vi "selectCursorProperties.vi"(6 "Cursor Properties in":T1={"Horizontal Line?"=TRUE, "Vertical Line?"=TRUE, "Timestamp"=enum."at BOTTOM", "time format (%H:%M:%S)"="%H:%M:%S", "size"=2, "font"={"Font Name"="Arial", "Size"=16, "Strikeout?"=FALSE, "Italic?"=FALSE, "Underline?"=FALSE, "Outline?"=FALSE, "Shadow"=FALSE, "Bold?"=FALSE}, "alignment(left, top)"={"Horizontal"=enum."center", "Vertical"=enum."center"}, "TextFormat"="%3$s\\n%2$.2f"} {"size" min=1 max=50}) -> (2 "ok":bool, 4 "Cursor Properties out":T1={"Horizontal Line?"=TRUE, "Vertical Line?"=TRUE, "Timestamp"=enum."at BOTTOM", "time format (%H:%M:%S)"="%H:%M:%S", "size"=2, "font"={"Font Name"="Arial", "Size"=16, "Strikeout?"=FALSE, "Italic?"=FALSE, "Underline?"=FALSE, "Outline?"=FALSE, "Shadow"=FALSE, "Bold?"=FALSE}, "alignment(left, top)"={"Horizontal"=enum."center", "Vertical"=enum."center"}, "TextFormat"="%3$s\\n%2$.2f"} {"size" min=1 max=50})   [LabVIEW 2017, in "QControl_Graph.lvclass"]
uses:
  QControl_Graph.lvclass
  Cursor Properties.ctl
  Font.ctl
  Alignment.ctl
  Alignment.Horizontal.ctl
  Alignment.Vertical.ctl
panel:
  in  "Y Label Vertical:":T5=enum."center"
  in  "Y Label Horizontal:":T4=enum."center"
  in  "Show Horizontal Lines":bool=TRUE
  in  "Show Vertical Lines":bool=TRUE
  in  "X Label Position:":enum16{"at TOP", "at BOTTOM", "none"}(ring)=enum."at BOTTOM"
  in  "Point Size:":i16=2 min=1 max=50
  in  "Time Format:":string
  in  "Name Format:":string
  in  "Bold":bool
  in  "Shadow":bool
  in  "Outline":bool
  in  "Strikeout":bool
  in  "Underline":bool
  in  "Italic":bool
  in  "Size :":i16
  in  "Font:":string
  in  "Cancel":bool
  in  "OK":bool
  # "Font"
  # "Effects"
  # "Cursor"
  # "Grid"
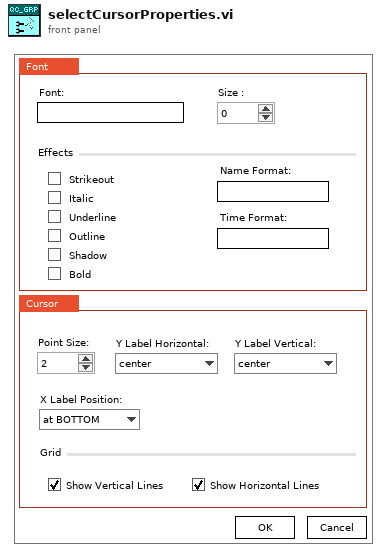
[diagram p1: front panel]
types:
  T1 = typedef "QControl_Graph.lvclass/Cursor Properties.ctl" = cluster{"Horizontal Line?":bool, "Vertical Line?":bool, "Timestamp":enum16{"at TOP", "at BOTTOM", "none"}, "time format (%H:%M:%S)":string, "size":i16, "font":T2, "alignment(left, top)":T3, "TextFormat":string}
  T2 = typedef "QControl_Graph.lvclass/Font.ctl" = cluster{"Font Name":string, "Size":i16, "Strikeout?":bool, "Italic?":bool, "Underline?":bool, "Outline?":bool, "Shadow":bool, "Bold?":bool}
  T3 = typedef "QControl_Graph.lvclass/Alignment.ctl" = cluster{"Horizontal":T4, "Vertical":T5}
  T4 = typedef "QControl_Graph.lvclass/Alignment.Horizontal.ctl" = enum16{"left", "center", "right"}
  T5 = typedef "QControl_Graph.lvclass/Alignment.Vertical.ctl" = enum16{"top", "center", "bottom"}
  T6 = enum32{"Invalid", "Standard", "Closed", "Hidden", "Minimized", "Maximized"}
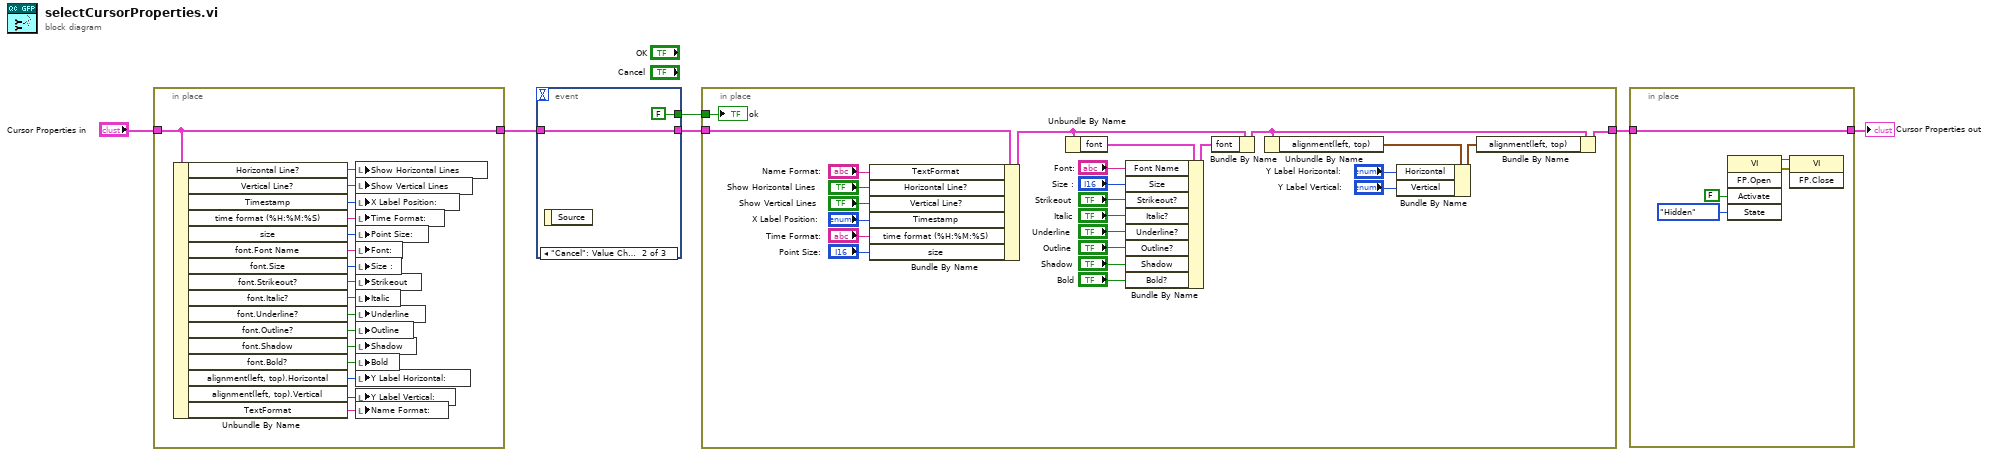
[diagram p0: block diagram]
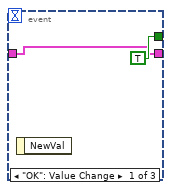
[diagram p2: hidden frame]
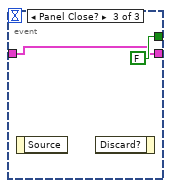
[diagram p3: hidden frame]
diagram:
  n1 = in-place {
    in-place-border: "Cursor Properties in" -> [w7]
    in-place-border: [w7] -> w5
    n2 = Unbundle By Name(w7) -> ("Horizontal Line?"=w23:bool, "Vertical Line?"=w22:bool, "Timestamp"=w21:enum16{"at TOP", "at BOTTOM", "none"}, "time format (%H:%M:%S)"=w20:string, "size"=w18:i16, "font.Font Name"=w19:string, "font.Size"=w17:i16, "font.Strikeout?"=w16:bool, "font.Italic?"=w8:bool, "font.Underline?"=w9:bool, "font.Outline?"=w10:bool, "font.Shadow"=w11:bool, "font.Bold?"=w12:bool, "alignment(left, top).Horizontal"=w15:T4, "alignment(left, top).Vertical"=w14:T5, "TextFormat"=w13:string)
    n3 = local write "Show Horizontal Lines"(w23) -> ()
    n4 = local write "Show Vertical Lines"(w22) -> ()
    n5 = local write "X Label Position:"(w21) -> ()
    n6 = local write "Time Format:"(w20) -> ()
    n7 = local write "Point Size:"(w18) -> ()
    n8 = local write "Font:"(w19) -> ()
    n9 = local write "Size :"(w17) -> ()
    n10 = local write "Strikeout"(w16) -> ()
    n11 = local write "Italic"(w8) -> ()
    n12 = local write "Underline"(w9) -> ()
    n13 = local write "Outline"(w10) -> ()
    n14 = local write "Shadow"(w11) -> ()
    n15 = local write "Bold"(w12) -> ()
    n16 = local write "Y Label Horizontal:"(w15) -> ()
    n17 = local write "Y Label Vertical:"(w14) -> ()
    n18 = local write "Name Format:"(w13) -> ()
  }
  n19 = event shown="[1] \"Cancel\": Value Change" {
    selector: _ -> [_ _ _]
    dyn-events: _ -> [_ _ _]
    timeout: _ -> [_ _ _]
    tunnel: [TRUE FALSE FALSE] -> w3
    tunnel: w5 -> [w24 w26 w28]
    tunnel: [w24 w26 w28] -> w4
    event "OK": Value Change {
      n20 = event-data() -> ()  [unwired: 1 in, 1 out]
    }
    event "Cancel": Value Change {
      n21 = event-data() -> ()  [unwired: 1 in, 1 out]
    }
    event Panel Close? {
      n22 = event-data() -> ()  [unwired: 1 in, 1 out]
      n23 = event-data() -> ()  [unwired: 2 in, 1 out]
    }
  }
  n24 = in-place {
    in-place-border: w4 -> [w48]
    in-place-border: [w31] -> w2
    in-place-border: w3 -> [w30]
    n25 = Bundle By Name(cluster=w48, "TextFormat"="Name Format:", "Horizontal Line?"="Show Horizontal Lines", "Vertical Line?"="Show Vertical Lines", "Timestamp"="X Label Position:", "time format (%H:%M:%S)"="Time Format:", "size"="Point Size:") -> (w38:T1)
    n26 = Unbundle By Name(w38) -> ("font"=w37:T2)
    n27 = Bundle By Name(cluster=w37, "Font Name"="Font:", "Size"="Size :", "Strikeout?"="Strikeout", "Italic?"="Italic", "Underline?"="Underline", "Outline?"="Outline", "Shadow"="Shadow", "Bold?"="Bold") -> (w47:T2)
    n28 = Bundle By Name(cluster=w38, "font"=w47) -> (w32:T1)
    n29 = Unbundle By Name(w32) -> ("alignment(left, top)"=w34:T3)
    n30 = Bundle By Name(cluster=w34, "Horizontal"="Y Label Horizontal:", "Vertical"="Y Label Vertical:") -> (w33:T3)
    n31 = Bundle By Name(cluster=w32, "alignment(left, top)"=w33) -> (w31:T1)
    "ok" <- w30
  }
  n32 = in-place {
    in-place-border: w2 -> [w55]
    in-place-border: [w55] -> w1
    n33 = invoke class="VI" method="FP.Open"("Activate"=FALSE ("Activate?"), "State"=T6."Hidden") -> (reference out=w57:refnum<vi>, error out=w59:errorcluster)  [unwired: 3 in, 3 out]
    n34 = invoke class="VI" method="FP.Close"(reference=w57, error in=w59) -> ()  [unwired: 1 in, 3 out]
  }
  "Cursor Properties out" <- w1
